vi "CSDB_Common.DB_entry_exists.vi"(5 "= (value)":string, 6 "select (coloumn)  (= ID)":string, 7 "error in (no error)":errorcluster, 8 "where (coloumn)":string, 9 "from (Table)":string, 10 "connection reference":T1) -> (0 "error out":errorcluster, 1 "first element":string, 2 "output array":string[](array[string]), 3 "connection reference out":T1, 4 "exists ?":bool)   [LabVIEW 2014, in "CSDB_Common.lvlib"]
uses:
  CSDB_Common.lvlib
  <vilib>/addons/database/Connection.llb/Conn ObjectReference.ctl
  <vilib>/addons/database/NI_Database_API.lvlib
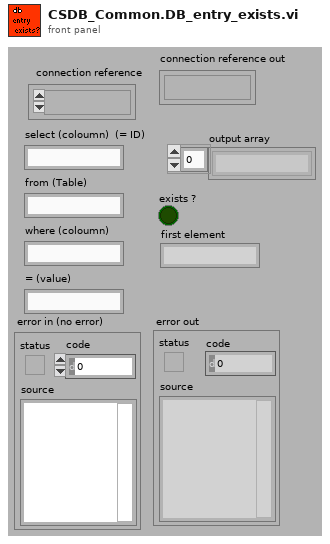
[diagram p1: front panel]
types:
  T1 = typedef "NI_Database_API.lvlib/Conn ObjectReference.ctl" = refnum<k1>
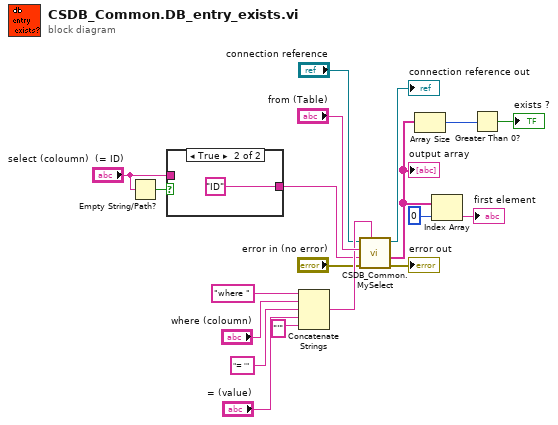
[diagram p0: block diagram]
diagram:
  n1 = Empty String/Path?(string/path="select (coloumn)  (= ID)") -> (empty?=w3:bool)
  n2 = case shown="True" w3 {
    tunnel: [w20 "ID"] -> w2
    tunnel: "select (coloumn)  (= ID)" -> [w20 _]
    frame False {
    }
    frame True {
    }
  }
  n3 = Concatenate Strings("where " ("string"), "where (coloumn)", "= '" ("string"), "= (value)", "'" ("string")) -> (w13:string)
  n4 = call "CSDB_Common.MySelect.vi"("optional clause"=w13, "error in (no error)"="error in (no error)", "column"=w2, "table"="from (Table)", "connection reference"="connection reference") -> ("error out"=→"error out":errorcluster, "1d output array"=w6:string[], "connection reference out"=→"connection reference out":T1)  [unwired: 2 in]
  "output array" <- w6
  n5 = Array Size(array=w6) -> (size(s)=w8:i32)
  n6 = Index Array(array=w6, index=0) -> (element=→"first element":string)
  n7 = Greater Than 0?(x=w8) -> (x > 0?=→"exists ?":bool)
